vi "configure.vi"(8 "error in (no error)":errorcluster, 11 "GenericPlugin in":refnum<class "ScanHeadAK130114ResonanceFlexRIO.lvclass">) -> (0 "error out":errorcluster, 3 "GenericPlugin out":refnum<class "ScanHeadAK130114ResonanceFlexRIO.lvclass">)   [LabVIEW 2010, in "ScanHeadAK130114ResonanceFlexRIO.lvclass"]
doc: "The dynamic dispatch version of this VI loads and displays the configuration file associated with the plug-in object. The user modify and save the configuration data."
uses:
  ScanHeadAK130114ResonanceFlexRIO.lvclass
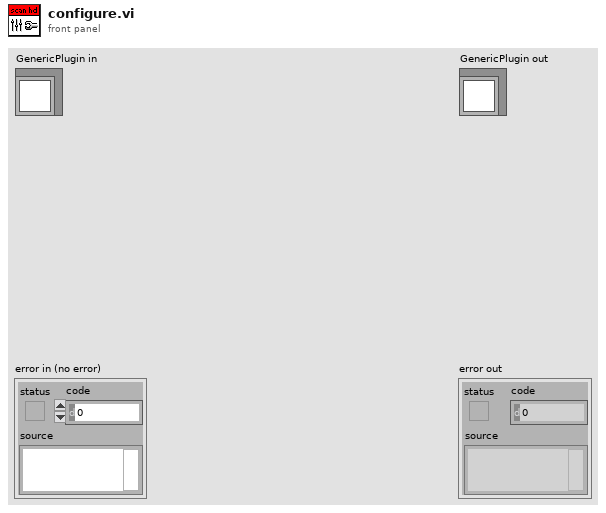
[diagram p1: front panel]
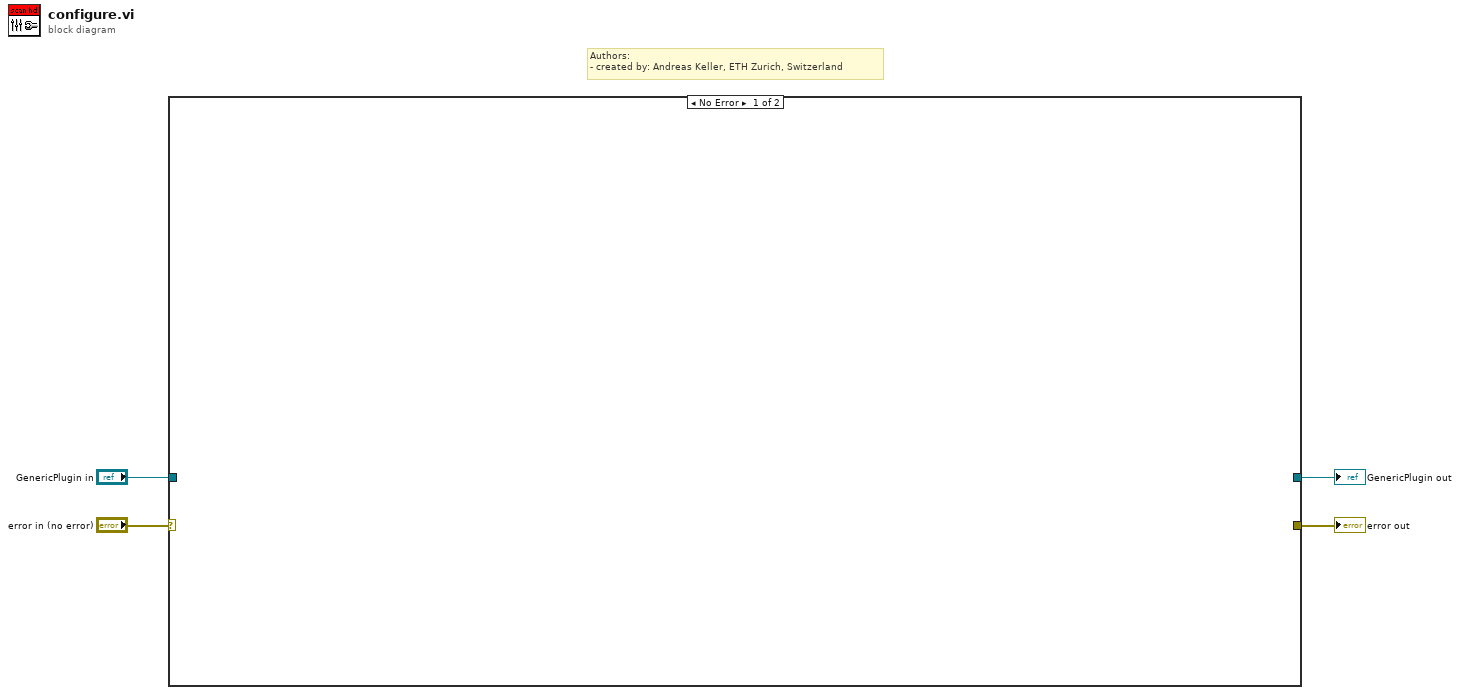
[diagram p0: block diagram]
diagram:
  # "Authors: \n- created by: Andreas Keller, ETH Zurich, Switzerland"
  n1 = case shown="No Error" "error in (no error)" {
    selector: "error in (no error)" -> [_ w6]
    tunnel: [_ w6] -> w3
    tunnel: [_ w5] -> w1
    tunnel: "GenericPlugin in" -> [_ w5]
    frame No Error {
    }
    frame Error {
    }
  }
  "error out" <- w3
  "GenericPlugin out" <- w1
